vi "ReadTextFiles2ExcelCSV.vi"() -> ()   [LabVIEW 2019]
uses:
  <vilib>/Utility/file.llb/Write Delimited Spreadsheet (string).vi
panel:
  in  "Run Number":string
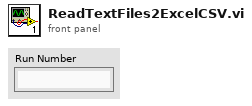
[diagram p1: front panel]
types:
  T1 = enum16{"open", "replace", "create", "open or create", "replace or create", "replace or create with confirmation"}
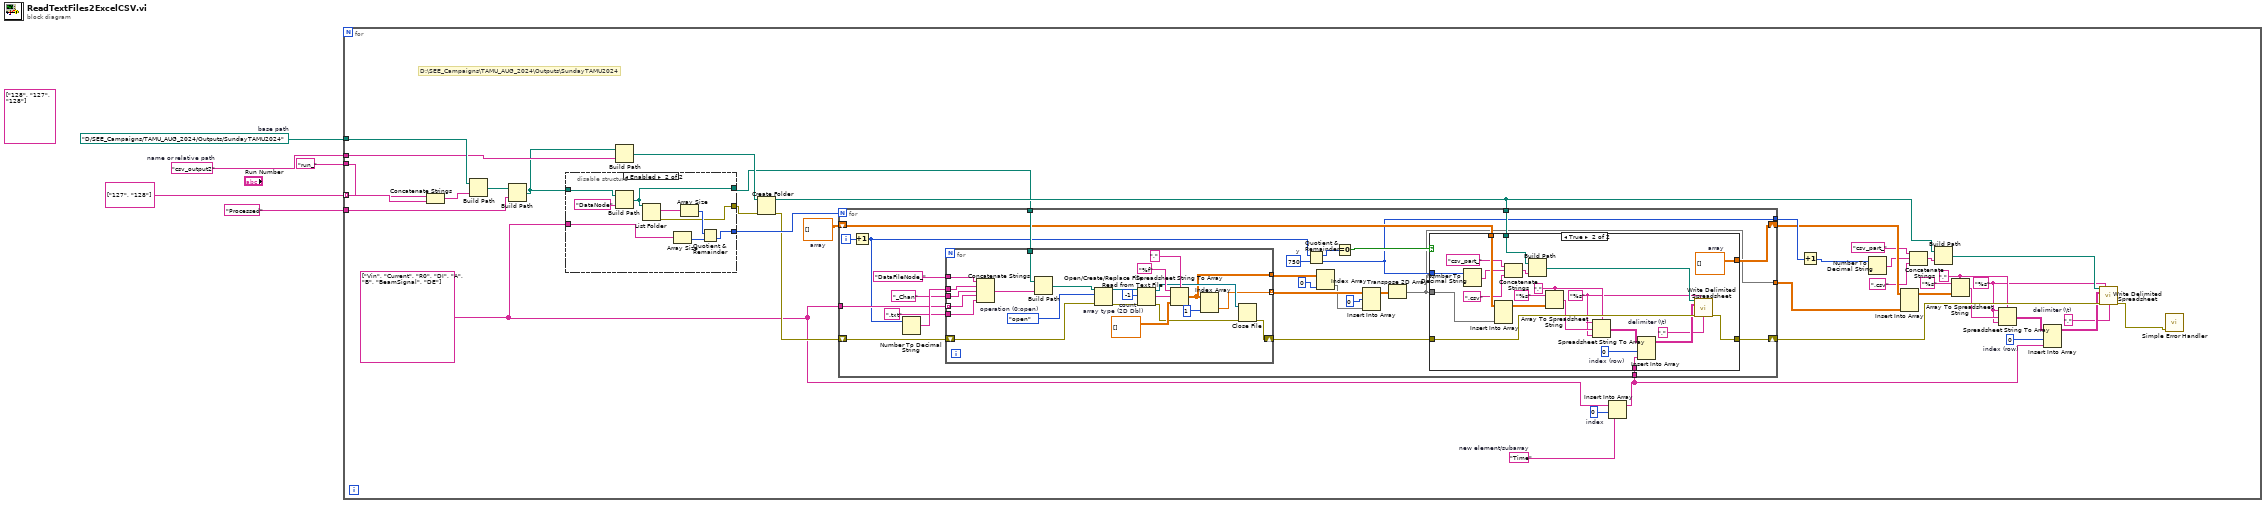
[diagram p0: block diagram]
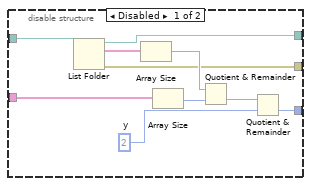
[diagram p2: hidden frame]
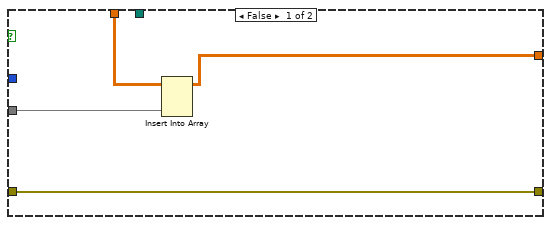
[diagram p3: hidden frame]
diagram:
  (unwired) string[] ["128", "127", "128"]
  w3 = "csv_output2"  # name or relative path
  w5 = path "D:/SEE_Campaigns/TAMU_AUG_2024/Outputs/SundayTAMU2024"  # base path
  n1 = for {
    tunnel: w5 -> [w12]
    tunnel: string[] ["127", "128"] -> [w11] mode=indexing
    tunnel: "run_" ("string") -> [w10]
    tunnel: w3 -> [w9]
    tunnel: "Processed" ("name or relative path") -> [w8]
    w14 = "Time"  # new element/subarray
    w15 = 0  # index
    w17 = ","  # delimiter (\t)
    w18 = 0  # index (row)
    w21 = "%s" ("format (%.3f)")
    w23 = "," ("delimiter (Tab)")
    w39 = dbl[][] []  # array
    w16 = string[] ["Vin", "Current", "R0", "DI", "A", "B", "BeamSignal", "DE"]
    # "D:\\SEE_Campaigns\\TAMU_AUG_2024\\Outputs\\SundayTAMU2024"
    n2 = Concatenate Strings(w10, w11) -> (w44:string)
    n3 = Build Path(base path=w12, name or relative path=w44) -> (appended path=w43:path)
    n4 = Build Path(base path=w43, name or relative path=w8) -> (appended path=w7:path)
    n5 = disable-structure shown="Enabled" {
      disable-tunnel: w7 -> [w51 w63]
      disable-tunnel: [w48 w57] -> w42
      disable-tunnel: [w47 w58] -> w41
      disable-tunnel: w16 -> [w46 w59]
      disable-tunnel: [w45 w55] -> w6
      frame Disabled {
        w49 = 2  # y
        n6 = List Folder(path=w51) -> (path out=w45:path, filenames=w54:string[], error out=w47:errorcluster)  [unwired: 3 in, 1 out]
        n7 = Array Size(array=w54) -> (size(s)=w52:i32)
        n8 = Array Size(array=w46) -> (size(s)=w53:i32)
        n9 = Quotient & Remainder(x=w52, y=w53) -> (floor(x/y)=w50:i32)  [unwired: 1 out]
        n10 = Quotient & Remainder(x=w50, y=w49) -> (floor(x/y)=w48:i32)  [unwired: 1 out]
      }
      frame Enabled {
        n11 = Build Path(base path=w63, name or relative path="DataNode") -> (appended path=w55:path)
        n12 = List Folder(path=w55) -> (filenames=w62:string[], error out=w58:errorcluster)  [unwired: 3 in, 2 out]
        n13 = Array Size(array=w59) -> (size(s)=w61:i32)
        n14 = Array Size(array=w62) -> (size(s)=w60:i32)
        n15 = Quotient & Remainder(x=w60, y=w61) -> (floor(x/y)=w57:i32)  [unwired: 1 out]
      }
    }
    n16 = Build Path(base path=w7, name or relative path=w9) -> (appended path=w38:path)
    n17 = Create Folder(path (use dialog)=w38, error in=w41) -> (created path=w32:path, error out=w40:errorcluster)  [unwired: 1 in, 1 out]
    n18 = Insert Into Array(array=w16, index=w15, new element=w14) -> (w13:string[])
    n19 = for {
      N: w42 -> [_]
      tunnel: w16 -> [w86]
      shift-right: [w70] -> w35
      shift-left: w40 -> [w83]
      tunnel: w6 -> [w84]
      shift-right: [w69] -> w34
      shift-left: w39 -> [w72]
      tunnel: w32 -> [w68]
      tunnel: w13 -> [w66]
      tunnel: [w65] -> w37
      tunnel: [w64] -> w33
      i -> [w77]
      w75 = 750  # y
      n20 = Increment(x=w77) -> (x+1=w76:i32)
      n21 = Number To Decimal String(number=w76) -> (decimal integer string=w89:string)  [unwired: 1 in]
      n22 = for {
        tunnel: w86 -> [w135] mode=indexing
        tunnel: w89 -> [w138]
        tunnel: "DataFileNode_" -> [w137]
        tunnel: "_Chan" -> [w136]
        tunnel: ".txt" ("string") -> [w134]
        tunnel: w84 -> [w132]
        shift-right: [w118] -> w71
        shift-left: w83 -> [w129]
        tunnel: [w117] -> w80 mode=indexing
        tunnel: [w116] -> w82
        w123 = dbl[][] []  # array type (2D Dbl)
        w126 = -1  # count
        w130 = T1."open"  # operation (0:open)
        n23 = Concatenate Strings(w137, w138, w136, w135, w134) -> (w133:string)
        n24 = Build Path(base path=w132, name or relative path=w133) -> (appended path=w131:path)
        n25 = Open/Create/Replace File(file path (use dialog)=w131, error in=w129, operation (0:open)=w130) -> (refnum out=w128:refnum<file>, error out=w127:errorcluster)  [unwired: 3 in, 1 out]
        n26 = Read from Text File(file (use dialog)=w128, count=w126, error in=w127) -> (refnum out=w120:refnum<file>, text=w125:string, error out=w119:errorcluster)  [unwired: 1 in, 1 out]
        n27 = Spreadsheet String To Array(delimiter (Tab)=",", format string="%f", spreadsheet string=w125, array type (2D Dbl)=w123) -> (array=w116:dbl[][])
        n28 = Index Array(array=w116, index (col)=1 ("disabled index (col)")) -> (element=w117:dbl[])  [unwired: 1 in]
        n29 = Close File(refnum=w120, error in=w119) -> (error out=w118:errorcluster)  [unwired: 1 out]
      }
      n30 = Quotient & Remainder(x=w76, y=w75) -> (x-y*floor(x/y)=w74:i32, floor(x/y)=w65:i32)
      n31 = Index Array(array=w82, index (col)=0 ("disabled index (col)")) -> (element=w79:dbl[])  [unwired: 1 in]
      n32 = Equal To 0?(x=w74) -> (x = 0?=w73:bool)
      n33 = Insert Into Array(array=w80, index (row)=0 ("disabled index (col)"), new element=w79) -> (w78:dbl[][])  [unwired: 1 in]
      n34 = Transpose 2D Array(2D array=w78) -> (transposed array=w64:dbl[][])
      n35 = case shown="True" w73 {
        tunnel: w64 -> [w92 w115]
        tunnel: w72 -> [w93 w114]
        tunnel: w65 -> [_ w110]
        tunnel: w71 -> [w91 w107]
        tunnel: [w91 w106] -> w70
        tunnel: [w90 w105] -> w69
        tunnel: w68 -> [_ w104]
        tunnel: w66 -> [_ w97]
        frame False {
          n36 = Insert Into Array(array=w93, new element=w92) -> (w90:dbl[][])  [unwired: 2 in]
        }
        frame True {
          w94 = ","  # delimiter (\t)
          w95 = 0  # index (row)
          w99 = "%s" ("format (%.3f)")
          w101 = "," ("delimiter (Tab)")
          w105 = dbl[][] []  # array
          n37 = Number To Decimal String(number=w110) -> (decimal integer string=w112:string)  [unwired: 1 in]
          n38 = Insert Into Array(array=w114, new element=w115) -> (w103:dbl[][])  [unwired: 2 in]
          n39 = Concatenate Strings("csv_part_", w112, ".csv") -> (w109:string)
          n40 = Build Path(base path=w104, name or relative path=w109) -> (appended path=w108:path)
          n41 = Array To Spreadsheet String(delimiter (Tab)=w101, array=w103, 3:"%s" ("format string")) -> (spreadsheet string=w100:string)
          n42 = Spreadsheet String To Array(delimiter (Tab)=w101, format string=w99, spreadsheet string=w100, array type (2D Dbl)=w99) -> (array=w98:string[][])
          n43 = Insert Into Array(array=w98, index (row)=w95, new element=w97) -> (w96:string[][])  [unwired: 1 in]
          n44 = call-poly <vilib>:"Write Delimited Spreadsheet.vi"("file path (dialog if empty)"=w108, "format (%s)"=w99, "2D data"=w96, "error in (no error)"=w107, "delimiter (\\t)"=w94) -> ("error out"=w106:errorcluster)  [unwired: 9 in, 1 out]
        }
      }
    }
    n45 = Increment(x=w37) -> (x+1=w36:i32)
    n46 = Number To Decimal String(number=w36) -> (decimal integer string=w29:string)  [unwired: 1 in]
    n47 = Insert Into Array(array=w34, new element=w33) -> (w25:dbl[][])  [unwired: 2 in]
    n48 = Concatenate Strings("csv_part_", w29, ".csv") -> (w27:string)
    n49 = Build Path(base path=w32, name or relative path=w27) -> (appended path=w26:path)
    n50 = Array To Spreadsheet String(delimiter (Tab)=w23, array=w25, 3:"%s" ("format string")) -> (spreadsheet string=w22:string)
    n51 = Spreadsheet String To Array(delimiter (Tab)=w23, format string=w21, spreadsheet string=w22, array type (2D Dbl)=w21) -> (array=w20:string[][])
    n52 = Insert Into Array(array=w20, index (row)=w18, new element=w13) -> (w19:string[][])  [unwired: 1 in]
    n53 = call-poly <vilib>:"Write Delimited Spreadsheet.vi"("file path (dialog if empty)"=w26, "format (%s)"=w21, "2D data"=w19, "error in (no error)"=w35, "delimiter (\\t)"=w17) -> ("error out"=w31:errorcluster)  [unwired: 9 in, 1 out]
    n54 = call <vilib>:"Simple Error Handler.vi"("error in (no error)"=w31) -> ()  [unwired: 4 in, 5 out]
  }
